vi "Element to Control.vi"(8 "error in (no error)":errorcluster, 10 "Element Type":string, 11 "Control List in":refnum<class "Control List.lvclass">) -> (0 "error out":errorcluster, 2 "Control Type":string, 3 "Control List out":refnum<class "Control List.lvclass">)   [LabVIEW 2020, in "VolatusGUIEditor.lvlib" / "Control List.lvclass"]
uses:
  Control List.lvclass
  Control List.lvclass/Control List.ctl
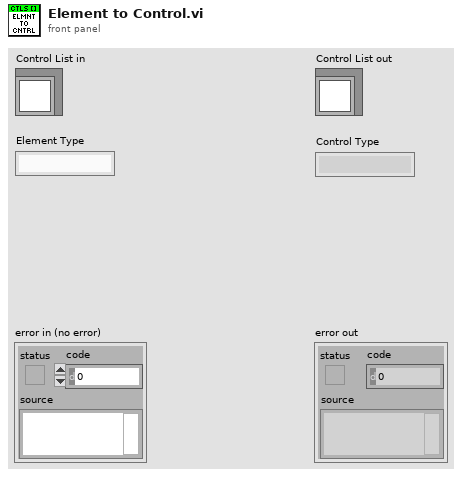
[diagram p1: front panel]
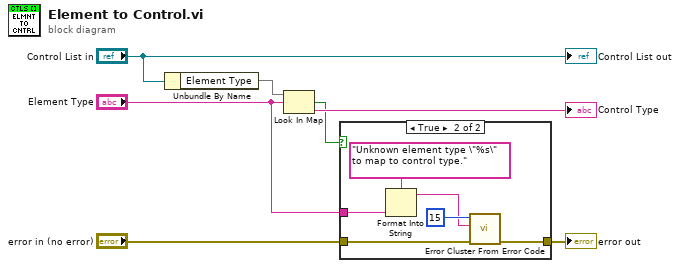
[diagram p0: block diagram]
diagram:
  n1 = Unbundle By Name("Control List in") -> ("Element Type"=w5:map{string, string})
  n2 = Look In Map(map=w5, key="Element Type") -> (key not found?=w2:bool, value=→"Control Type":string)  [unwired: 1 in]
  n3 = case shown="True" w2 {
    tunnel: "error in (no error)" -> [w8 w14]
    tunnel: [w8 w13] -> w3
    tunnel: "Element Type" -> [_ w9]
    frame False {
    }
    frame True {
      n4 = Format Into String(format string="Unknown element type \"%s\" to map to control type.", w9) -> (resulting string=w11:string)  [unwired: 2 in, 1 out]
      n5 = call <vilib>:"Error Cluster From Error Code.vi"("error in (no error)"=w14, "error message (\"\")"=w11, "error code (0)"=15) -> ("error out"=w13:errorcluster)  [unwired: 6 in]
    }
  }
  "error out" <- w3
  "Control List out" <- "Control List in"
